vi "Test Cannot Open View Before Start.vi"(8 "error in (no error)":errorcluster, 11 "View Test In":refnum<class "View Test.lvclass">) -> (0 "error out":errorcluster, 3 "View Test Out":refnum<class "View Test.lvclass">)   [LabVIEW 2020, in "View Test.lvclass"]
uses:
  View Test.lvclass
  C:/Program Files (x86)/National Instruments/LabVIEW 2020/vi.lib/Astemes/LUnit/Test Case.lvclass
  Framework/Process/Process.lvclass/Process.ctl
  Framework/View/View.lvclass/View.ctl
  <vilib>/Astemes/LUnit/Test Case.lvclass/Test Case.ctl
  <vilib>/Astemes/LUnit/LUnit Assertion Result.lvclass/LUnit Assertion Result.ctl
  <vilib>/Astemes/LUnit/LUnit Test Case Result.lvclass/LUnit Test Case Result.ctl
  <vilib>/Astemes/LUnit/LUnit Method Result.lvclass/LUnit Method Result.ctl
  Framework/Process/Protected/Messaging/Enqueue Message.vi
  Framework/View/Public/Get View VI Reference.vi
  Framework/Process/Public/Lifecycle/Get Lifecycle State.vi
  <vilib>/Astemes/LUnit/Palette/Fail.vi
  <vilib>/Astemes/LUnit/Palette/Pass.vi
  <vilib>/Astemes/LUnit/Set Assertion Type.vi
  Framework/Process/Protected/Messaging/Request Message.vi
  <vilib>/Utility/error.llb/Clear Errors.vi
  <vilib>/Astemes/LUnit/Add test result.vi
  <vilib>/Astemes/LUnit/LUnit Write Passed.vi
  <vilib>/Astemes/LUnit/LUnit Write Message.vi
  <vilib>/Astemes/LUnit/LUnit Write Description.vi
  <vilib>/Astemes/LUnit/LUnit Write Assertion Type.vi
  Framework/Process/Private/SubVIs/Enqueue Request Message.vi
  <vilib>/Astemes/LUnit/LUnit Record Assertion Result.vi
  <vilib>/Astemes/LUnit/LUnit Aggregate Assertion Results.vi
  <vilib>/Astemes/LUnit/Assertion Result/LUnit Read Status.vi
  <vilib>/Astemes/LUnit/LUnit Read Message.vi
  <vilib>/Astemes/LUnit/LUnit Read Description.vi
  <vilib>/Astemes/LUnit/Method Result/LUnit Merge Status.vi
  <vilib>/Astemes/LUnit/LUnit Concatenate result strings.vi
  Framework/View/View.lvclass
  C:/Users/anton/Documents/GitHub/Triarc-Framework/source/Framework/Process/Process.lvclass
  <vilib>/Utility/error.llb/Error Cluster From Error Code.vi
  Framework/Process/Private/SubVIs/Wait for Response Message.vi
  <vilib>/Astemes/LUnit/LUnit Assertion Result.lvclass
  View Test.lvclass/View Test.ctl
  <vilib>/Astemes/LUnit/Test Case.lvclass
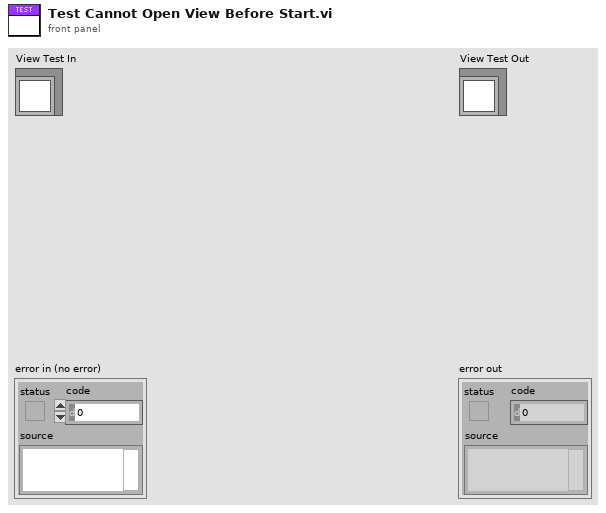
[diagram p1: front panel]
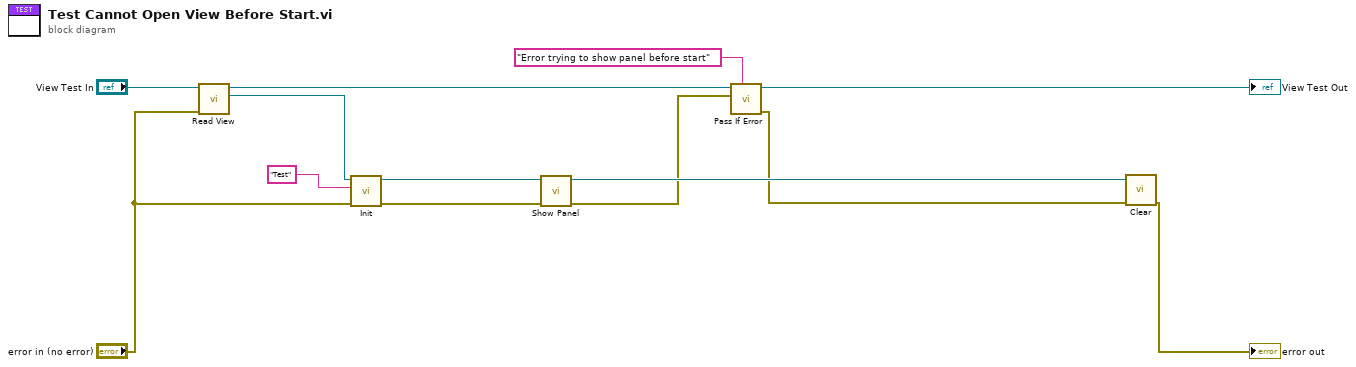
[diagram p0: block diagram]
diagram:
  n1 = call "Read View.vi"("error in (no error)"="error in (no error)", "View Test In"="View Test In") -> ("View"=w12:refnum<class "View.lvclass">, "View Test Out"=w13:refnum<class "View Test.lvclass">)  [unwired: 7 in, 1 out]
  n2 = call-dynamic "Init.vi"("error in (no error)"="error in (no error)", "Name"="Test", "View In"=w12) -> ("error out"=w6:errorcluster, "View Out"=w7:refnum<class "View.lvclass">)  [unwired: 7 in]
  n3 = call "Show Panel.vi"("error in (no error)"=w6, "View In"=w7) -> ("error out"=w3:errorcluster, "View Out"=w5:refnum<class "View.lvclass">)  [unwired: 8 in]
  n4 = call <vilib>:"Pass If Error.vi"("Description"="Error trying to show panel before start", "Assert error"=w3, "LUnit Test Case In"=w13) -> ("error out"=w1:errorcluster, "LUnit Test Case Out"=→"View Test Out":refnum<class "View Test.lvclass">)  [unwired: 7 in]
  n5 = call-dynamic "Clear.vi"("error in (no error)"=w1, "View In"=w5) -> ("error out"=→"error out":errorcluster)  [unwired: 9 in]
